vi "LV SET REGISTER.vi"(8 "error in (no error)":errorcluster, 9 "Board Handle In":T1, 10 "Value":u32, 11 "Name":string) -> (0 "error out":errorcluster, 1 "Board Handle Out":T1, 3 "NI Error Code":i32)   [LabVIEW 2021]
uses:
  SciSDK_Labview.lvlib
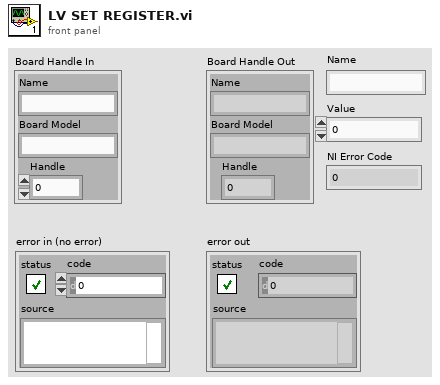
[diagram p1: front panel]
types:
  T1 = cluster{"Name":string, "Board Model":string, "Handle":u64}
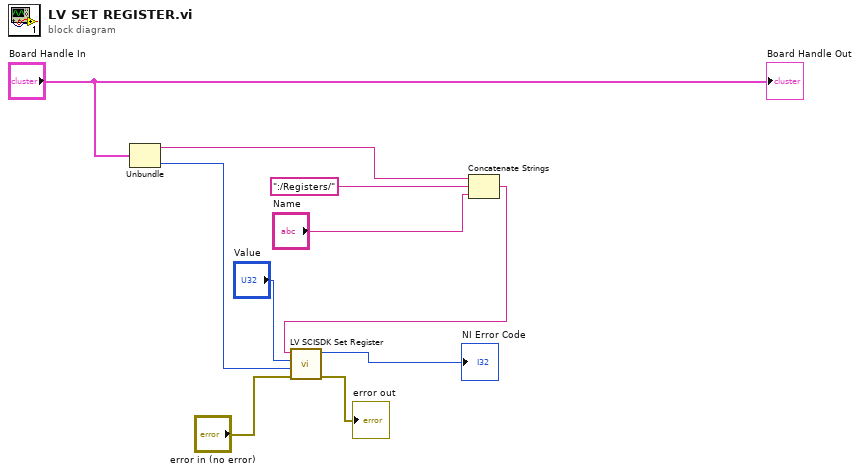
[diagram p0: block diagram]
diagram:
  n1 = Unbundle("Board Handle In") -> ("Name"=w7:string, "Handle"=w9:u64)  [unwired: 1 out]
  n2 = Concatenate Strings(w7, ":/Registers/" ("string"), "Name") -> (w5:string)
  n3 = call "LV SCISDK Set Register.vi"("error in (no error)"="error in (no error)", "handle"=w9, "value"="Value", "Path"=w5) -> ("error out"=→"error out":errorcluster, "function return"=→"NI Error Code":i32)  [unwired: 5 in, 1 out]
  "Board Handle Out" <- "Board Handle In"
